vi "ReqRep.vi"() -> ()   [LabVIEW 2025]
uses:
  libzmq-v143-mt-4_3_6/ctls/SocketType.ctl
  zeromq/Receive_string.vi
  zeromq/Send_string.vi
  zeromq/Context.lvclass
  libzmq-v143-mt-4_3_6/LibZMQ.lvlib
  zeromq/Socket.lvclass
panel:
  out "Routed back 4":string
  out "Routed back 3":string
  out "error out 3":errorcluster
  out "error out (should error)":errorcluster
  out "Routed back 2":string
  out "error out 2":errorcluster
  out "error out":errorcluster
  out "Routed back":string
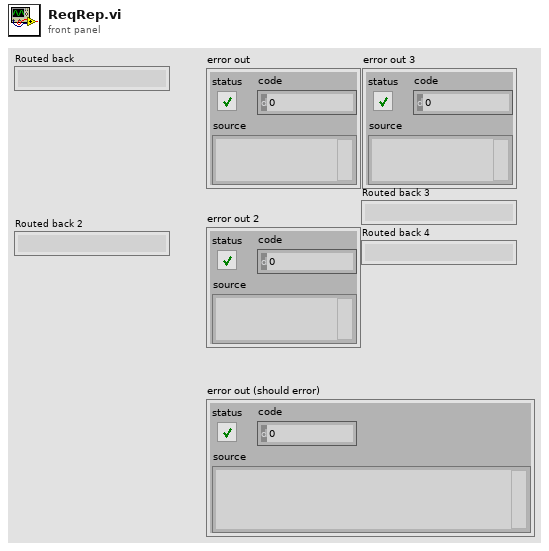
[diagram p1: front panel]
types:
  T1 = typedef "LibZMQ.lvlib/SocketType.ctl" = enum8{"PAIR", "PUB", "SUB", "REQ", "REP", "DEALER", "ROUTER", "PULL", "PUSH", "XPUB", "XSUB", "STREAM"}
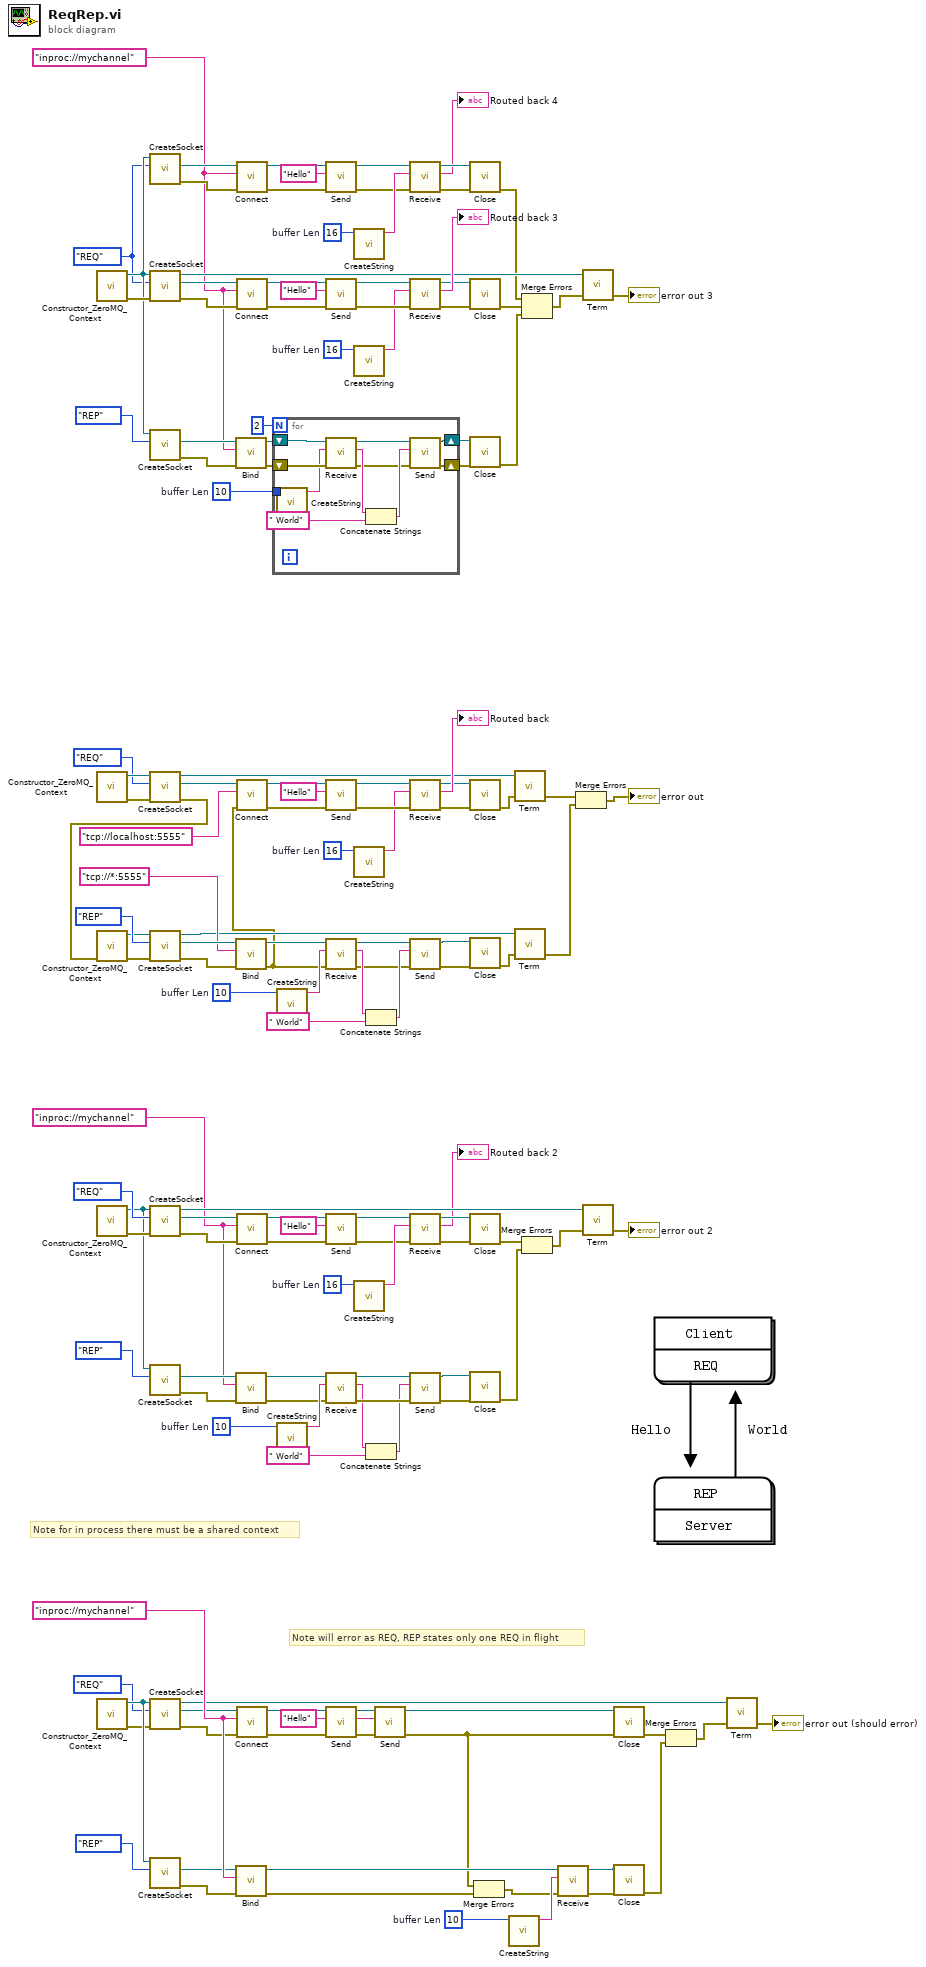
[diagram p0: block diagram]
diagram:
  w9 = 16  # buffer Len
  w30 = 16  # buffer Len
  w36 = 10  # buffer Len
  w4 = SocketType."REQ" ("Socket Type")
  w3 = "inproc://mychannel"
  w63 = 16  # buffer Len
  w74 = 10  # buffer Len
  w92 = "Hello" ("data")
  w101 = 10  # buffer Len
  w107 = "inproc://mychannel"
  w134 = 16  # buffer Len
  w122 = 10  # buffer Len
  w116 = "inproc://mychannel"
  # "Note will error as REQ, REP states only one REQ in flight"
  # "Note for in process there must be a shared context"
  n1 = call "Constructor_ZeroMQ_Context.vi"() -> ("error out"=w40:errorcluster, "context out"=w5:refnum<class "Context.lvclass">)  [unwired: 10 in]
  n2 = call "Constructor_ZeroMQ_Context.vi"() -> ("error out"=w82:errorcluster, "context out"=w83:refnum<class "Context.lvclass">)  [unwired: 10 in]
  n3 = call "Constructor_ZeroMQ_Context.vi"() -> ("error out"=w117:errorcluster, "context out"=w115:refnum<class "Context.lvclass">)  [unwired: 10 in]
  n4 = call "Constructor_ZeroMQ_Context.vi"() -> ("error out"=w106:errorcluster, "context out"=w108:refnum<class "Context.lvclass">)  [unwired: 10 in]
  n5 = call "CreateSocket.vi"("Socket Type"=w4, "context in"=w5) -> ("error out"=w14:errorcluster, "socket out"=w12:refnum<class "Socket.lvclass">)  [unwired: 7 in, 1 out]
  n6 = call "CreateSocket.vi"("error in"=w40, "Socket Type"=w4, "context in"=w5) -> ("error out"=w25:errorcluster, "socket out"=w27:refnum<class "Socket.lvclass">, "context out"=w21:refnum<class "Context.lvclass">)  [unwired: 6 in]
  n7 = call "CreateSocket.vi"("Socket Type"=SocketType."REP", "context in"=w5) -> ("error out"=w37:errorcluster, "socket out"=w38:refnum<class "Socket.lvclass">)  [unwired: 7 in, 1 out]
  n8 = call "CreateSocket.vi"("error in"=w82, "Socket Type"=SocketType."REQ", "context in"=w83) -> ("error out"=w44:errorcluster, "socket out"=w60:refnum<class "Socket.lvclass">, "context out"=w54:refnum<class "Context.lvclass">)  [unwired: 6 in]
  n9 = call "Constructor_ZeroMQ_Context.vi"("error in"=w44) -> ("error out"=w79:errorcluster, "context out"=w78:refnum<class "Context.lvclass">)  [unwired: 9 in]
  n10 = call "CreateSocket.vi"("error in"=w79, "Socket Type"=SocketType."REP", "context in"=w78) -> ("error out"=w75:errorcluster, "socket out"=w77:refnum<class "Socket.lvclass">, "context out"=w48:refnum<class "Context.lvclass">)  [unwired: 6 in]
  n11 = call "CreateSocket.vi"("error in"=w117, "Socket Type"=SocketType."REQ", "context in"=w115) -> ("error out"=w139:errorcluster, "socket out"=w137:refnum<class "Socket.lvclass">, "context out"=w143:refnum<class "Context.lvclass">)  [unwired: 6 in]
  n12 = call "CreateSocket.vi"("Socket Type"=SocketType."REP", "context in"=w115) -> ("error out"=w121:errorcluster, "socket out"=w120:refnum<class "Socket.lvclass">)  [unwired: 7 in, 1 out]
  n13 = call "CreateSocket.vi"("error in"=w106, "Socket Type"=SocketType."REQ", "context in"=w108) -> ("error out"=w96:errorcluster, "socket out"=w98:refnum<class "Socket.lvclass">, "context out"=w94:refnum<class "Context.lvclass">)  [unwired: 6 in]
  n14 = call "CreateSocket.vi"("Socket Type"=SocketType."REP", "context in"=w108) -> ("error out"=w102:errorcluster, "socket out"=w103:refnum<class "Socket.lvclass">)  [unwired: 7 in, 1 out]
  n15 = call "Bind.vi"("error in"=w37, "endpoint"=w3, "socket in"=w38) -> ("error out"=w34:errorcluster, "socket out"=w35:refnum<class "Socket.lvclass">)  [unwired: 7 in]
  n16 = call "Bind.vi"("error in"=w75, "endpoint"="tcp://*:5555", "socket in"=w77) -> ("error out"=w45:errorcluster, "socket out"=w73:refnum<class "Socket.lvclass">)  [unwired: 7 in]
  n17 = call "Bind.vi"("error in"=w121, "endpoint"=w116, "socket in"=w120) -> ("error out"=w124:errorcluster, "socket out"=w123:refnum<class "Socket.lvclass">)  [unwired: 7 in]
  n18 = call "Bind.vi"("error in"=w102, "endpoint"=w107, "socket in"=w103) -> ("error out"=w89:errorcluster, "socket out"=w100:refnum<class "Socket.lvclass">)  [unwired: 7 in]
  n19 = call "Connect.vi"("error in"=w14, "endpoint"=w3, "socket in"=w12) -> ("error out"=w15:errorcluster, "socket out"=w13:refnum<class "Socket.lvclass">)  [unwired: 7 in]
  n20 = call "Connect.vi"("error in"=w25, "endpoint"=w3, "socket in"=w27) -> ("error out"=w24:errorcluster, "socket out"=w26:refnum<class "Socket.lvclass">)  [unwired: 7 in]
  n21 = call "Connect.vi"("error in"=w45, "endpoint"="tcp://localhost:5555", "socket in"=w60) -> ("error out"=w57:errorcluster, "socket out"=w59:refnum<class "Socket.lvclass">)  [unwired: 7 in]
  n22 = call "Connect.vi"("error in"=w139, "endpoint"=w116, "socket in"=w137) -> ("error out"=w140:errorcluster, "socket out"=w138:refnum<class "Socket.lvclass">)  [unwired: 7 in]
  n23 = call "Connect.vi"("error in"=w96, "endpoint"=w107, "socket in"=w98) -> ("error out"=w95:errorcluster, "socket out"=w97:refnum<class "Socket.lvclass">)  [unwired: 7 in]
  n24 = for {
    N: 2 -> [_]
    tunnel: w36 -> [w157]
    shift-right: [w148] -> w20
    shift-left: w35 -> [w156]
    shift-right: [w147] -> w19
    shift-left: w34 -> [w155]
    n25 = call "CreateString.vi"("length"=w157) -> ("string"=w154:string)  [unwired: 10 in]
    n26 = call-poly "Receive.vi"("error in"=w155, "buf in"=w154, "socket in"=w156) -> ("error out"=w149:errorcluster, "data"=w152:string, "socket out"=w153:refnum<class "Socket.lvclass">)  [unwired: 6 in]
    n27 = Concatenate Strings(w152, " World") -> (w150:string)
    n28 = call-poly "Send.vi"("error in"=w149, "data"=w150, "socket in"=w153) -> ("error out"=w147:errorcluster, "socket out"=w148:refnum<class "Socket.lvclass">)  [unwired: 7 in]
  }
  n29 = call "CreateString.vi"("length"=w74) -> ("string"=w72:string)  [unwired: 10 in]
  n30 = call "CreateString.vi"("length"=w122) -> ("string"=w125:string)  [unwired: 10 in]
  n31 = call-poly "Send.vi"("error in"=w15, "data"="Hello", "socket in"=w13) -> ("error out"=w8:errorcluster, "socket out"=w7:refnum<class "Socket.lvclass">)  [unwired: 7 in]
  n32 = call-poly "Send.vi"("error in"=w24, "data"="Hello", "socket in"=w26) -> ("error out"=w31:errorcluster, "socket out"=w32:refnum<class "Socket.lvclass">)  [unwired: 7 in]
  n33 = call-poly "Send.vi"("error in"=w57, "data"="Hello", "socket in"=w59) -> ("error out"=w64:errorcluster, "socket out"=w65:refnum<class "Socket.lvclass">)  [unwired: 7 in]
  n34 = call-poly "Receive.vi"("error in"=w45, "buf in"=w72, "socket in"=w73) -> ("error out"=w67:errorcluster, "data"=w70:string, "socket out"=w71:refnum<class "Socket.lvclass">)  [unwired: 6 in]
  n35 = call-poly "Send.vi"("error in"=w140, "data"="Hello", "socket in"=w138) -> ("error out"=w133:errorcluster, "socket out"=w132:refnum<class "Socket.lvclass">)  [unwired: 7 in]
  n36 = call-poly "Receive.vi"("error in"=w124, "buf in"=w125, "socket in"=w123) -> ("error out"=w130:errorcluster, "data"=w127:string, "socket out"=w126:refnum<class "Socket.lvclass">)  [unwired: 6 in]
  n37 = call-poly "Send.vi"("error in"=w95, "data"=w92, "socket in"=w97) -> ("error out"=w90:errorcluster, "socket out"=w91:refnum<class "Socket.lvclass">)  [unwired: 7 in]
  n38 = call "CreateString.vi"("length"=w9) -> ("string"=w10:string)  [unwired: 10 in]
  n39 = call "CreateString.vi"("length"=w30) -> ("string"=w29:string)  [unwired: 10 in]
  n40 = call "CreateString.vi"("length"=w63) -> ("string"=w62:string)  [unwired: 10 in]
  n41 = call "CreateString.vi"("length"=w134) -> ("string"=w135:string)  [unwired: 10 in]
  n42 = Concatenate Strings(w70, " World") -> (w68:string)
  n43 = Concatenate Strings(w127, " World") -> (w129:string)
  n44 = call-poly "Send.vi"("error in"=w90, "data"=w92, "socket in"=w91) -> ("error out"=w86:errorcluster, "socket out"=w85:refnum<class "Socket.lvclass">)  [unwired: 7 in]
  n45 = call-poly "Receive.vi"("error in"=w8, "buf in"=w10, "socket in"=w7) -> ("error out"=w17:errorcluster, "data"=→"Routed back 4":string, "socket out"=w16:refnum<class "Socket.lvclass">)  [unwired: 6 in]
  n46 = call-poly "Receive.vi"("error in"=w31, "buf in"=w29, "socket in"=w32) -> ("error out"=w22:errorcluster, "data"=→"Routed back 3":string, "socket out"=w23:refnum<class "Socket.lvclass">)  [unwired: 6 in]
  n47 = call-poly "Receive.vi"("error in"=w64, "buf in"=w62, "socket in"=w65) -> ("error out"=w55:errorcluster, "data"=→"Routed back":string, "socket out"=w56:refnum<class "Socket.lvclass">)  [unwired: 6 in]
  n48 = call-poly "Send.vi"("error in"=w67, "data"=w68, "socket in"=w71) -> ("error out"=w49:errorcluster, "socket out"=w50:refnum<class "Socket.lvclass">)  [unwired: 7 in]
  n49 = call-poly "Receive.vi"("error in"=w133, "buf in"=w135, "socket in"=w132) -> ("error out"=w142:errorcluster, "data"=→"Routed back 2":string, "socket out"=w141:refnum<class "Socket.lvclass">)  [unwired: 6 in]
  n50 = call-poly "Send.vi"("error in"=w130, "data"=w129, "socket in"=w126) -> ("error out"=w145:errorcluster, "socket out"=w144:refnum<class "Socket.lvclass">)  [unwired: 7 in]
  n51 = call "Close.vi"("error in"=w17, "socket"=w16) -> ("error out"=w2:errorcluster)  [unwired: 9 in]
  n52 = call "Close.vi"("error in"=w22, "socket"=w23) -> ("error out"=w41:errorcluster)  [unwired: 9 in]
  n53 = call "Close.vi"("error in"=w19, "socket"=w20) -> ("error out"=w18:errorcluster)  [unwired: 9 in]
  n54 = call "Close.vi"("error in"=w55, "socket"=w56) -> ("error out"=w53:errorcluster)  [unwired: 9 in]
  n55 = call "Close.vi"("error in"=w49, "socket"=w50) -> ("error out"=w51:errorcluster)  [unwired: 9 in]
  n56 = call "Close.vi"("error in"=w142, "socket"=w141) -> ("error out"=w114:errorcluster)  [unwired: 9 in]
  n57 = call "Close.vi"("error in"=w145, "socket"=w144) -> ("error out"=w146:errorcluster)  [unwired: 9 in]
  n58 = Merge Errors(w86, w89) -> (w88:errorcluster)
  n59 = call "CreateString.vi"("length"=w101) -> ("string"=w99:string)  [unwired: 10 in]
  n60 = call "Term.vi"("error in"=w53, "context in"=w54) -> ("error out"=w52:errorcluster)  [unwired: 3 in]
  n61 = call "Term.vi"("error in"=w51, "context in"=w48) -> ("error out"=w47:errorcluster)  [unwired: 3 in]
  n62 = Merge Errors(w2, w41, w18) -> (w42:errorcluster)
  n63 = Merge Errors(w114, w146) -> (w113:errorcluster)
  n64 = call-poly "Receive.vi"("error in"=w88, "buf in"=w99, "socket in"=w100) -> ("error out"=w87:errorcluster, "socket out"=w84:refnum<class "Socket.lvclass">)  [unwired: 6 in, 1 out]
  n65 = Merge Errors(w52, w47) -> (→"error out":errorcluster)
  n66 = call "Term.vi"("error in"=w42, "context in"=w21) -> ("error out"=→"error out 3":errorcluster)  [unwired: 3 in]
  n67 = call "Term.vi"("error in"=w113, "context in"=w143) -> ("error out"=→"error out 2":errorcluster)  [unwired: 3 in]
  n68 = call "Close.vi"("error in"=w86, "socket"=w85) -> ("error out"=w109:errorcluster)  [unwired: 9 in]
  n69 = call "Close.vi"("error in"=w87, "socket"=w84) -> ("error out"=w93:errorcluster)  [unwired: 9 in]
  n70 = Merge Errors(w109, w93) -> (w110:errorcluster)
  n71 = call "Term.vi"("error in"=w110, "context in"=w94) -> ("error out"=→"error out (should error)":errorcluster)  [unwired: 3 in]
